vi "FPGA SPI_Write Read.vi"(7 "Total Bits":u16=8, 8 "error in":errorcluster, 9 "Write Data":u8[](array[numeric]), 10 "Port (0)":u8, 11 "FPGA VI Reference":T1) -> (0 "error out":errorcluster, 2 "Read Data":u8[](array[numeric]), 3 "FPGA VI Reference Out":T1)   [LabVIEW 2012]
uses:
  Controls/FPGA SPI_FPGA Ref.ctl
  FPGA/Controls/FPGA SPI_Cmd.ctl
  <vilib>/Utility/error.llb/Error Cluster From Error Code.vi
  <vilib>/rvi/errors/niLvFpgaAdjustHostInterfaceError.vi
  <vilib>/rvi/interface/nirviReadWriteControl/nirviReadWriteControl.xnode
  FPGA Bitfiles/Whirlybird_FPGATarget_WhirlybirdFPGAMa_DBA2D843.lvbitx
  Whirlybird FPGA Main.vi
  NiFpgaLv.dll
panel:
  out "Numeric":i32
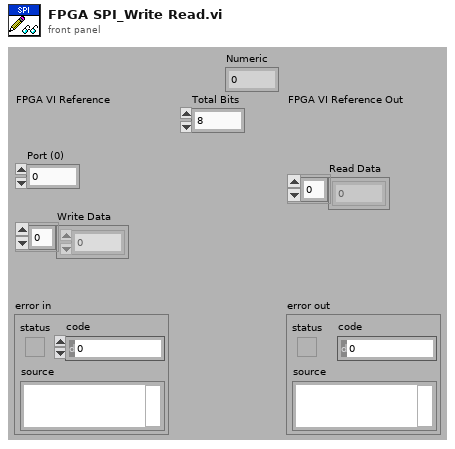
[diagram p1: front panel]
types:
  T1 = typedef "FPGA SPI_FPGA Ref.ctl" = refnum<k20>
  T2 = enum16{"Start", "Write", "Read", "Wait Until Done"}
  T3 = typedef "FPGA SPI_Cmd.ctl" = enum8{"Idle", "Write/Read SPI", "Configure"}
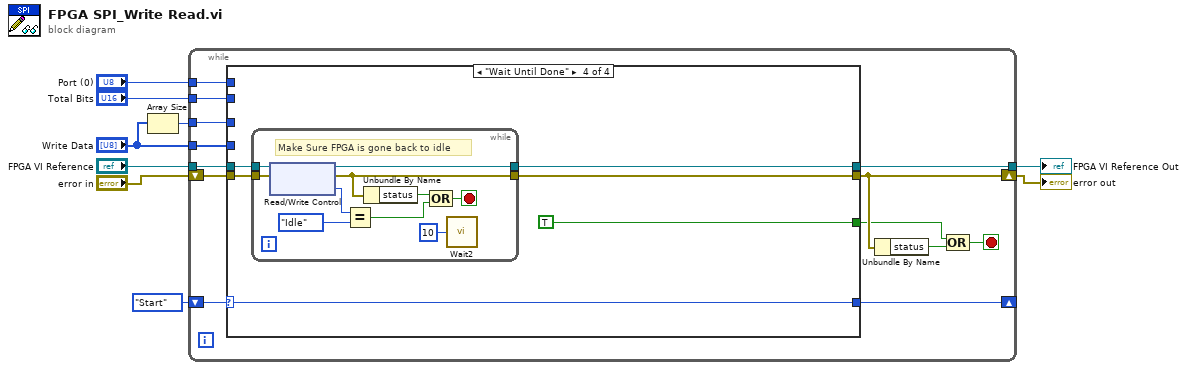
[diagram p0: block diagram]
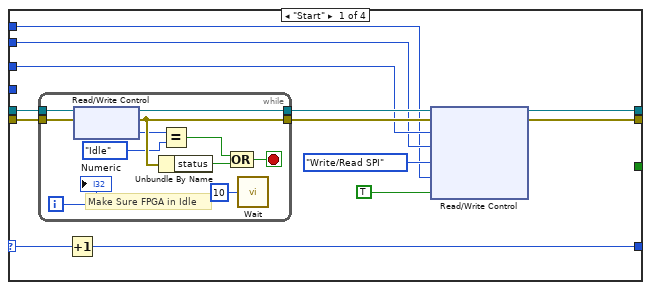
[diagram p2: hidden frame]
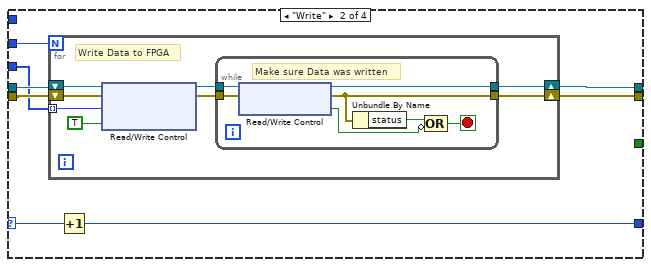
[diagram p3: hidden frame]
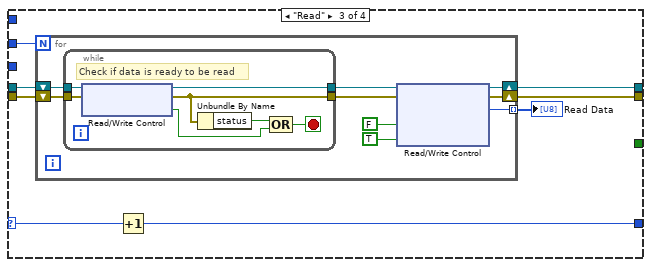
[diagram p4: hidden frame]
diagram:
  n1 = Array Size(array="Write Data") -> (size(s)=w8:i32)
  n2 = while {
    tunnel: "FPGA VI Reference" -> [w22]
    tunnel: w8 -> [w20]
    tunnel: "Write Data" -> [w19]
    tunnel: [w18] -> w6
    shift-right: [w17] -> w5
    shift-left: "error in" -> [w21]
    shift-right: [w12] -> _
    shift-left: T2."Start" -> [w13]
    tunnel: "Total Bits" -> [w11]
    tunnel: "Port (0)" -> [w10]
    stop <- w14 stop-if-true
    n3 = case shown="\"Wait Until Done\"" w13 {
      selector: w13 -> [w24 w47 w71 w95]
      tunnel: w22 -> [w33 w54 w76 w99]
      tunnel: w21 -> [w32 w53 w75 w98]
      tunnel: w20 -> [w31 w52 w74 _]
      tunnel: w19 -> [_ w51 _ _]
      tunnel: [w29 w49 w73 w97] -> w18
      tunnel: [w30 w50 w72 w96] -> w17
      tunnel: [_ _ _ TRUE] -> w16
      tunnel: [w23 w48 w70 w95] -> w12
      tunnel: w11 -> [w27 _ _ _]
      tunnel: w10 -> [w25 _ _ _]
      frame "Start" {
        n4 = while {
          tunnel: w33 -> [w46]
          tunnel: [w45] -> w35
          tunnel: w32 -> [w44]
          tunnel: [w41] -> w34
          i -> [w36]
          stop <- w42 stop-if-true
          # "Make Sure FPGA in Idle"
          n5 = xnode "Read/Write Control"("FPGA VI Reference In"=w46, "error in"=w44) -> ("FPGA VI Reference Out"=w45:T1, "error out"=w41:errorcluster, "SPI_Cmd"=w38:T3)
          n6 = Unbundle By Name(w41) -> ("status"=w43:bool)
          n7 = Equal?(x=w38, y=FPGA_SPI_Cmd."Idle" ("Type")) -> (x = y?=w39:bool)
          n8 = Compound Arithmetic op=OR(w39, w43) -> (w42:bool)
          n9 = call "Wait"("Count(uSec)"=u32 10 ("millisecond multiple")) -> ()  [unwired: 1 out]
          "Numeric" <- w36
        }
        n10 = Increment(x=w24) -> (x+1=w23:T2)
        n11 = xnode "Read/Write Control"("FPGA VI Reference In"=w35, "error in"=w34, "SPI_Total Bytes"=w31, "SPI_Total Bits"=w27, "SPI_Cmd"=FPGA_SPI_Cmd."Write/Read SPI" ("Cmd"), "SPI_Port"=w25, "SPI_Start"=TRUE ("Start")) -> ("FPGA VI Reference Out"=w29:T1, "error out"=w30:errorcluster)
      }
      frame "Write" {
        n12 = for {
          N: w52 -> [_]
          shift-right: [w56] -> w49
          shift-left: w54 -> [w62]
          shift-right: [w55] -> w50
          shift-left: w53 -> [w61]
          tunnel: w51 -> [w58] mode=indexing
          # "Write Data to FPGA"
          n13 = xnode "Read/Write Control"("FPGA VI Reference In"=w62, "error in"=w61, "SPI_Write Data"=w58, "SPI_Write Flag"=TRUE ("Write Flag")) -> ("FPGA VI Reference Out"=w60:T1, "error out"=w59:errorcluster)
          n14 = while {
            tunnel: w60 -> [w69]
            tunnel: w59 -> [w68]
            tunnel: [w67] -> w56
            tunnel: [w66] -> w55
            stop <- w63 stop-if-true
            # "Make sure Data was written"
            n15 = xnode "Read/Write Control"("FPGA VI Reference In"=w69, "error in"=w68) -> ("FPGA VI Reference Out"=w67:T1, "error out"=w66:errorcluster, "SPI_Write Flag"=w64:bool)
            n16 = Unbundle By Name(w66) -> ("status"=w65:bool)
            n17 = Compound Arithmetic op=OR(w65, invert w64) -> (w63:bool)
          }
        }
        n18 = Increment(x=w47) -> (x+1=w48:T2)
      }
      frame "Read" {
        n19 = for {
          N: w74 -> [_]
          shift-right: [w82] -> w73
          shift-left: w76 -> [w86]
          shift-right: [w81] -> w72
          shift-left: w75 -> [w85]
          tunnel: [w80] -> w77 mode=indexing
          n20 = while {
            tunnel: w86 -> [w88]
            tunnel: w85 -> [w93]
            tunnel: [w92] -> w84
            tunnel: [w91] -> w83
            stop <- w89 stop-if-true
            # "Check if data is ready to be read"
            n21 = xnode "Read/Write Control"("FPGA VI Reference In"=w88, "error in"=w93) -> ("FPGA VI Reference Out"=w92:T1, "error out"=w91:errorcluster, "SPI_Read Flag"=w87:bool)
            n22 = Unbundle By Name(w91) -> ("status"=w90:bool)
            n23 = Compound Arithmetic op=OR(w90, w87) -> (w89:bool)
          }
          n24 = xnode "Read/Write Control"("FPGA VI Reference In"=w84, "error in"=w83, "SPI_Read Flag"=FALSE ("Read Flag"), "SPI_Ack Read"=TRUE ("Write Flag")) -> ("FPGA VI Reference Out"=w82:T1, "error out"=w81:errorcluster, "SPI_Read Data"=w80:u8)
        }
        "Read Data" <- w77
        n25 = Increment(x=w71) -> (x+1=w70:T2)
      }
      frame "Wait Until Done" {
        n26 = while {
          tunnel: w99 -> [w109]
          tunnel: [w108] -> w97
          tunnel: w98 -> [w107]
          tunnel: [w104] -> w96
          stop <- w101 stop-if-true
          # "Make Sure FPGA is gone back to idle"
          n27 = xnode "Read/Write Control"("FPGA VI Reference In"=w109, "error in"=w107) -> ("FPGA VI Reference Out"=w108:T1, "error out"=w104:errorcluster, "SPI_Cmd"=w106:T3)
          n28 = Equal?(x=w106, y=FPGA_SPI_Cmd."Idle") -> (x = y?=w102:bool)
          n29 = Unbundle By Name(w104) -> ("status"=w103:bool)
          n30 = Compound Arithmetic op=OR(w103, w102) -> (w101:bool)
          n31 = call "Wait2"("Count(uSec)"=u32 10 ("millisecond multiple")) -> ()  [unwired: 1 out]
        }
      }
    }
    n32 = Unbundle By Name(w17) -> ("status"=w15:bool)
    n33 = Compound Arithmetic op=OR(w16, w15) -> (w14:bool)
  }
  "FPGA VI Reference Out" <- w6
  "error out" <- w5
